vi "Shot Type Selector.vi"(9 "Key?":bool, 10 "Distance?":bool) -> (2 "Shot Type":T1)   [LabVIEW 2016]
uses:
  Common Code/Shot Type.ctl
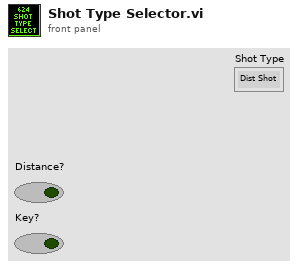
[diagram p1: front panel]
types:
  T1 = typedef "Shot Type.ctl" = enum16{"Dist Shot", "Key Shot"}
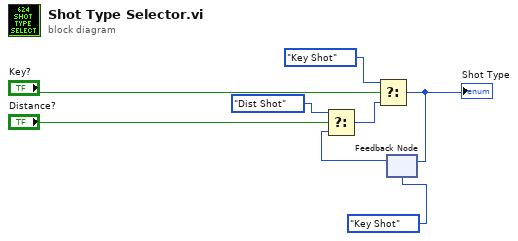
[diagram p0: block diagram]
diagram:
  n1 = feedback #1(Shot_Type."Key Shot" ("Shot Type")) -> (w1:T1)
  n2 = Select(t=Shot_Type."Dist Shot" ("Shot Type"), s="Distance?", f=w1) -> (s? t:f=w6:T1)
  n3 = Select(t=Shot_Type."Key Shot" ("Shot Type"), s="Key?", f=w6) -> (s? t:f=w2:T1)
  "Shot Type" <- w2
  n4 = feedback-in #1(w2) -> ()
